vi "Configure Offset and Limits (Spectrum Emission Mask - RBW).vi"(0 "VISA resource name":refnum<visa-resource-name>, 1 "Auto Sweep Time List":bool[](array[boolean])=[TRUE, TRUE, TRUE, TRUE, TRUE, TRUE], 2 "Auto Resolution Bandwidth List":bool[](array[boolean])=[FALSE, FALSE, FALSE, FALSE, FALSE, FALSE], 5 "Device Mode (1: BTS)":i32(ring)=1 items=["BTS"=1, "MS"=2], 7 "Manual Resolution Bandwidth List":dbl[](array[numeric])=[30000.0, 30000.0, 30000.0, 30000.0, 30000.0, 30000.0] format="%#.6g", 9 "Measurement Bandwidth List":i32[](array[numeric])=[1, 1, 1, 1, 1, 1] format="%.0g", 11 "error in (no error)":errorcluster, 12 "Manual Sweep Time List":dbl[](array[numeric])=[0.0173, 0.0173, 0.0173, 0.0173, 0.0173, 0.0173] format="%#.6g") -> (4 "VISA resource name out":refnum<visa-resource-name>, 15 "error out":errorcluster)   [LabVIEW 2014, in "Agilent MXA Series.lvlib"]
doc: "Configures the RBW settings under the offsets and limits for Spectrum Emission Mask measurement type."
uses:
  Agilent MXA Series.lvlib
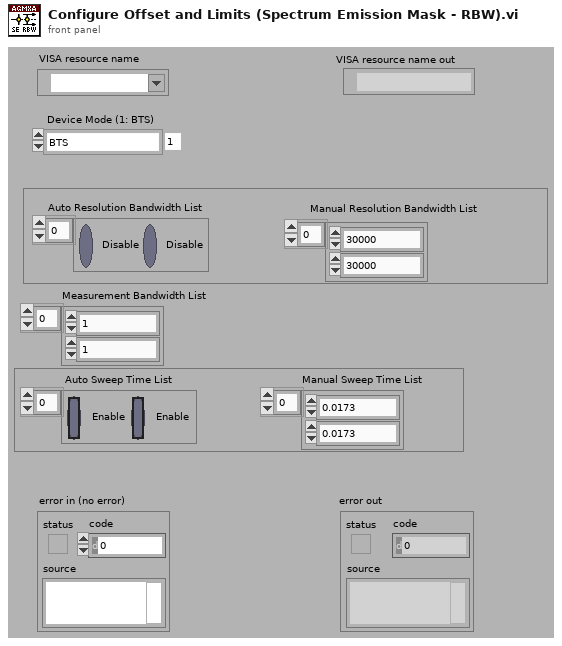
[diagram p1: front panel]
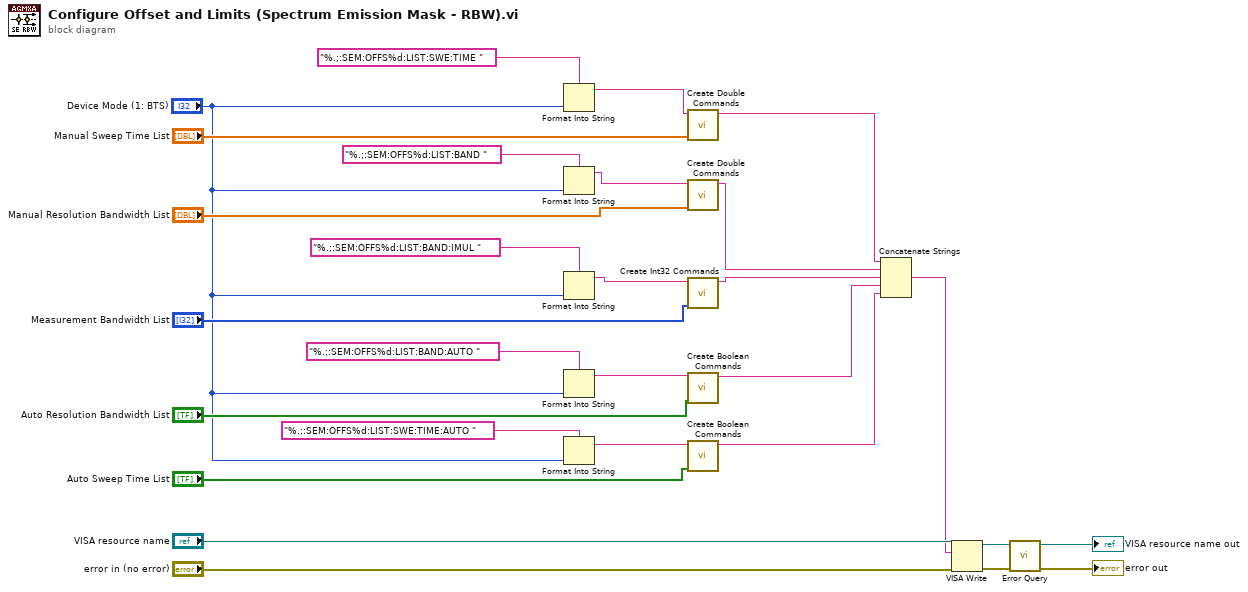
[diagram p0: block diagram]
diagram:
  n1 = Format Into String(format string="%.;:SEM:OFFS%d:LIST:SWE:TIME ", "Device Mode (1: BTS)") -> (resulting string=w26:string)  [unwired: 2 in, 1 out]
  n2 = Format Into String(format string="%.;:SEM:OFFS%d:LIST:BAND ", "Device Mode (1: BTS)") -> (resulting string=w24:string)  [unwired: 2 in, 1 out]
  n3 = Format Into String(format string="%.;:SEM:OFFS%d:LIST:BAND:IMUL ", "Device Mode (1: BTS)") -> (resulting string=w21:string)  [unwired: 2 in, 1 out]
  n4 = Format Into String(format string="%.;:SEM:OFFS%d:LIST:BAND:AUTO ", "Device Mode (1: BTS)") -> (resulting string=w18:string)  [unwired: 2 in, 1 out]
  n5 = Format Into String(format string="%.;:SEM:OFFS%d:LIST:SWE:TIME:AUTO ", "Device Mode (1: BTS)") -> (resulting string=w14:string)  [unwired: 2 in, 1 out]
  n6 = call "Create Double Commands.vi"("Double Values"="Manual Sweep Time List", "Commands"=w26) -> ("Result"=w4:string)  [unwired: 9 in]
  n7 = call "Create Double Commands.vi"("Double Values"="Manual Resolution Bandwidth List", "Commands"=w24) -> ("Result"=w3:string)  [unwired: 9 in]
  n8 = call "Create Int32 Commands.vi"("Int Values"="Measurement Bandwidth List", "Commands"=w21) -> ("Result"=w13:string)  [unwired: 9 in]
  n9 = call "Create Boolean Commands.vi"("Boolean States"="Auto Resolution Bandwidth List", "Command"=w18) -> ("Result String"=w12:string)  [unwired: 9 in]
  n10 = call "Create Boolean Commands.vi"("Boolean States"="Auto Sweep Time List", "Command"=w14) -> ("Result String"=w11:string)  [unwired: 9 in]
  n11 = Concatenate Strings(w4, w3, w13, w12, w11) -> (w2:string)
  n12 = VISA Write(VISA resource name="VISA resource name", write buffer=w2, error in (no error)="error in (no error)") -> (VISA resource name out=w9:refnum<visa-resource-name>, error out=w8:errorcluster)  [unwired: 1 out]
  n13 = call "Error Query.vi"("error in (no error)"=w8, "VISA resource name"=w9) -> ("error out"=→"error out":errorcluster, "VISA resource name out"=→"VISA resource name out":refnum<visa-resource-name>)  [unwired: 6 in, 2 out]
